vi "Initialise Front Panel.vi"(7 "This VI":refnum<vi>, 11 "UI Ref":T1) -> (0 "error out":errorcluster)   [LabVIEW 2021]
uses:
  Controls/UI References.ctl
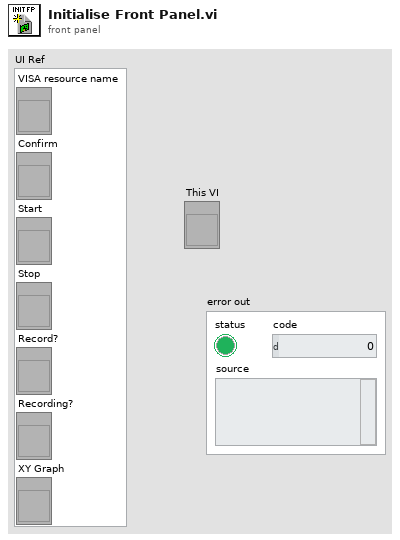
[diagram p1: front panel]
types:
  T1 = typedef "UI References.ctl" = cluster{"VISA resource name":refnum<vi>, "Confirm":refnum<vi>, "Start":refnum<vi>, "Stop":refnum<vi>, "Record?":refnum<vi>, "Recording?":refnum<vi>, "XY Graph":refnum<vi>}
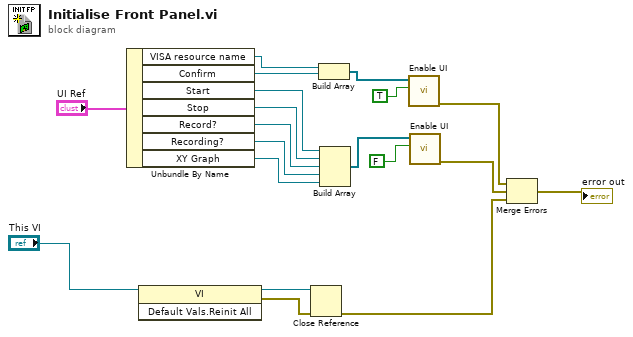
[diagram p0: block diagram]
diagram:
  n1 = Unbundle By Name("UI Ref") -> ("VISA resource name"=w1:refnum<vi>, "Confirm"=w2:refnum<vi>, "Start"=w9:refnum<vi>, "Stop"=w8:refnum<vi>, "Record?"=w7:refnum<vi>, "Recording?"=w6:refnum<vi>, "XY Graph"=w5:refnum<vi>)
  n2 = invoke class="VI" method="Default Vals.Reinit All"(reference="This VI") -> (reference out=w18:refnum<vi>, error out=w17:errorcluster)  [unwired: 2 in, 1 out]
  n3 = Close Reference(reference=w18, error in (no error)=w17) -> (error out=w14:errorcluster)
  n4 = Build Array(w1, w2) -> (w4:refnum<vi>[])
  n5 = Build Array(w9, w8, w7, w6, w5) -> (w3:refnum<vi>[])
  n6 = call "Enable UI.vi"("Enable?"=TRUE, "output cluster"=w4) -> ("error out"=w12:errorcluster)  [unwired: 9 in]
  n7 = call "Enable UI.vi"("Enable?"=FALSE, "output cluster"=w3) -> ("error out"=w10:errorcluster)  [unwired: 9 in]
  n8 = Merge Errors(w12, w10, w14) -> (→"error out":errorcluster)
